vi "Test Assert Less.vi"(8 "error in (no error)":errorcluster) -> (0 "error out":errorcluster)   [LabVIEW 2013]
uses:
  classes/Assert/Assert.lvclass
  classes/Test/Test.lvclass
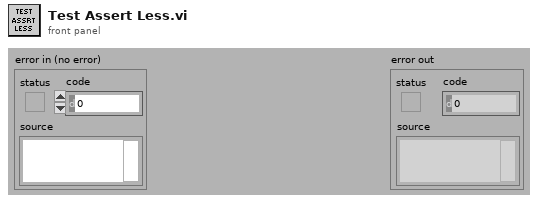
[diagram p1: front panel]
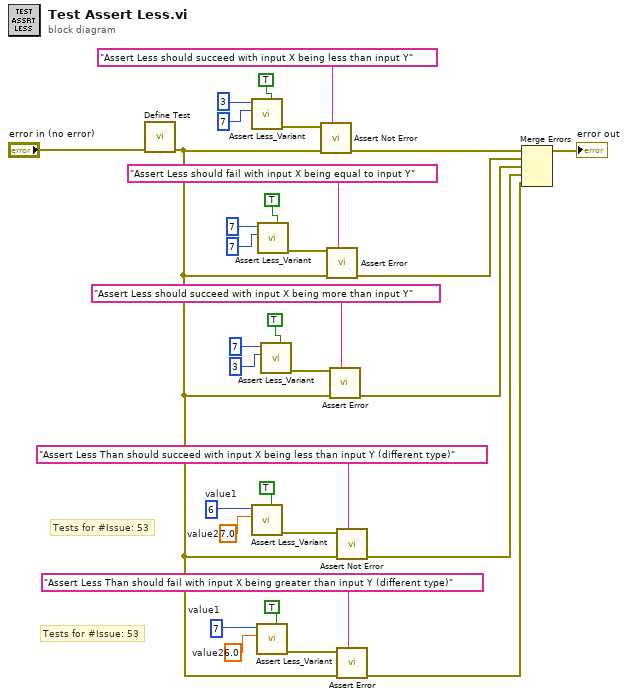
[diagram p0: block diagram]
diagram:
  w6 = 6.0  # value2
  w5 = 7  # value1
  w11 = 7.0  # value2
  w12 = 6  # value1
  # "Tests for #Issue: 53"
  # "Tests for #Issue: 53"
  n1 = call "Define Test.vi"("error in (no error)"="error in (no error)") -> ("error out"=w2:errorcluster)  [unwired: 10 in]
  n2 = call "Assert Less_Variant.vi"("Assert Only? (F)"=TRUE, "Y"=7, "X"=3) -> ("error out"=w33:errorcluster)  [unwired: 8 in]
  n3 = call "Assert Less_Variant.vi"("Assert Only? (F)"=TRUE, "Y"=w11, "X"=w12) -> ("error out"=w10:errorcluster)  [unwired: 8 in]
  n4 = call "Assert Less_Variant.vi"("Assert Only? (F)"=TRUE, "Y"=w6, "X"=w5) -> ("error out"=w3:errorcluster)  [unwired: 8 in]
  n5 = call "Assert Less_Variant.vi"("Assert Only? (F)"=TRUE, "Y"=7, "X"=7) -> ("error out"=w31:errorcluster)  [unwired: 8 in]
  n6 = call "Assert Less_Variant.vi"("Assert Only? (F)"=TRUE, "Y"=3, "X"=7) -> ("error out"=w19:errorcluster)  [unwired: 8 in]
  n7 = call "Assert Not Error.vi"("Label"="Assert Less should succeed with input X being less than input Y", "error in (no error)"=w2, "Not Error?"=w33) -> ("error out"=w25:errorcluster)  [unwired: 8 in]
  n8 = call "Assert Error.vi"("Label"="Assert Less should fail with input X being equal to input Y", "error in (no error)"=w2, "Error?"=w31) -> ("error out"=w26:errorcluster)  [unwired: 8 in]
  n9 = call "Assert Error.vi"("Label"="Assert Less should succeed with input X being more than input Y", "error in (no error)"=w2, "Error?"=w19) -> ("error out"=w14:errorcluster)  [unwired: 8 in]
  n10 = call "Assert Not Error.vi"("Label"="Assert Less Than should succeed with input X being less than input Y (different type)", "error in (no error)"=w2, "Not Error?"=w10) -> ("error out"=w9:errorcluster)  [unwired: 8 in]
  n11 = call "Assert Error.vi"("Label"="Assert Less Than should fail with input X being greater than input Y (different type)", "error in (no error)"=w2, "Error?"=w3) -> ("error out"=w4:errorcluster)  [unwired: 8 in]
  n12 = Merge Errors(w25, w26, w14, w9, w4) -> (→"error out":errorcluster)
